vi "GeoData.vi"() -> ()   [LabVIEW 2017] (continued)
AL\tMontgomery County\tH1\n36131\t1101\tMontgomery\tAL\tMontgomery County\tH1\n36054\t1101\tMillbrook\tAL\tMontgomery County\tH1\n36109\t1101\tMontgomery\tAL\tMontgomery County\tH1\n36041\t1101\tHighland home\tAL\tMontgomery County\tH1\n36107\t1101\tMontgomery\tAL\tMontgomery County\tH1\n36121\t1101\tMontgomery\tAL\tMontgomery County\tH1\n36117\t1101\tMontgomery\tAL\tMontgomery County\tH1\n36120\t1101\tMontgomery\tAL\tMontgomery County\tH1\n36123\t1101\tMontgomery\tAL\tMontgomery County\tH1\n36064\t1101\tPike road\tAL\tMontgomery County\tH1\n36105\t1101\tMontgomery\tAL\tMontgomery County\tH1\n36106\t1101\tMontgomery\tAL\tMontgomery County\tH1\n36116\t1101\tMontgomery\tAL\tMontgomery County\tH1\n36119\t1101\tMontgomery\tAL\tMontgomery County\tH1\n36065\t1101\tPine level\tAL\tMontgomery County\tH1\n36036\t1101\tGrady\tAL\tMontgomery County\tH1\n36046\t1101\tLapine\tAL\tMontgomery County\tH1\n36057\t1101\tMount meigs\tAL\tMontgomery County\tH1\n35175\t1103\tUnion grove\tAL\tMorgan County\tH1\n35619\t1103\tDanville\tAL\tMorgan County\tH1\n35640\t1103\tHartselle\tAL\tMorgan County\tH1\n35602\t1103\tDecatur\tAL\tMorgan County\tH1\n35058\t1103\tCullman\tAL\tMorgan County\tH1\n35601\t1103\tDecatur\tAL\tMorgan County\tH1\n35087\t1103\tJoppa\tAL\tMorgan County\tH1\n35673\t1103\tTrinity\tAL\tMorgan County\tH1\n35775\t1103\tValhermoso springs\tAL\tMorgan County\tH1\n35603\t1103\tDecatur\tAL\tMorgan County\tH1\n35019\t1103\tBaileyton\tAL\tMorgan County\tH1\n35016\t1103\tArab\tAL\tMorgan County\tH1\n35754\t1103\tLaceys spring\tAL\tMorgan County\tH1\n35179\t1103\tVinemont\tAL\tMorgan County\tH1\n35621\t1103\tEva\tAL\tMorgan County\tH1\n35622\t1103\tFalkville\tAL\tMorgan County\tH1\n35670\t1103\tSomerville\tAL\tMorgan County\tH1\n36786\t1105\tUniontown\tAL\tPerry County\tH1\n36756\t1105\tMarion\tAL\tPerry County\tH1\n36773\t1105\tSafford\tAL\tPerry County\tH1\n36701\t1105\tSelma\tAL\tPerry County\tH1\n35042\t1105\tCentreville\tAL\tPerry County\tH1\n36765\t1105\tNewbern\tAL\tPerry County\tH1\n36728\t1105\tCatherine\tAL\tPerry County\tH1\n35034\t1105\tBrent\tAL\tPerry County\tH1\n36759\t1105\tMarion junction\tAL\tPerry County\tH1\n36793\t1105\tLawley\tAL\tPerry County\tH1\n35576\t1107\tMillport\tAL\tPickens County\tH1\n35466\t1107\tGordo\tAL\tPickens County\tH1\n35447\t1107\tCarrollton\tAL\tPickens County\tH1\n35471\t1107\tMc shan\tAL\tPickens County\tH1\n35481\t1107\tReform\tAL\tPickens County\tH1\n35442\t1107\tAliceville\tAL\tPickens County\tH1\n35461\t1107\tEthelsville\tAL\tPickens County\tH1\n35574\t1107\tKennedy\tAL\tPickens County\tH1\n35555\t1107\tFayette\tAL\tPickens County\tH1\n36082\t1109\tTroy\tAL\tPike County\tH1\n36079\t1109\tTroy\tAL\tPike County\tH1\n36081\t1109\tTroy\tAL\tPike County\tH1\n36049\t1109\tLuverne\tAL\tPike County\tH1\n36010\t1109\tBrundidge\tAL\tPike County\tH1\n36034\t1109\tGlenwood\tAL\tPike County\tH1\n36035\t1109\tGoshen\tAL\tPike County\tH1\n36005\t1109\tBanks\tAL\tPike County\tH1\n36264\t1111\tHeflin\tAL\tRandolph County\tH1\n36266\t1111\tLineville\tAL\tRandolph County\tH1\n36258\t1111\tDelta\tAL\tRandolph County\tH1\n36278\t1111\tWedowee\tAL\tRandolph County\tH1\n36263\t1111\tGraham\tAL\tRandolph County\tH1\n36276\t1111\tWadley\tAL\tRandolph County\tH1\n36280\t1111\tWoodland\tAL\tRandolph County\tH1\n36274\t1111\tRoanoke\tAL\tRandolph County\tH1\n36874\t1113\tSalem\tAL\tRussell County\tH1\n36871\t1113\tPittsview\tAL\tRussell County\tH1\n36877\t1113\tSmiths station\tAL\tRussell County\tH1\n36804\t1113\tOpelika\tAL\tRussell County\tH1\n36869\t1113\tPhenix city\tAL\tRussell County\tH1\n36860\t1113\tHurtsboro\tAL\tRussell County\tH1\n36875\t1113\tSeale\tAL\tRussell County\tH1\n36856\t1113\tFort mitchell\tAL\tRussell County\tH1\n36053\t1113\tMidway\tAL\tRussell County\tH1\n36858\t1113\tHatchechubbee\tAL\tRussell County\tH1\n36868\t1113\tPhenix city\tAL\tRussell County\tH1\n36851\t1113\tCottonton\tAL\tRussell County\tH1\n36027\t1113\tEufaula\tAL\tRussell County\tH1\n36867\t1113\tPhenix city\tAL\tRussell County\tH1\n36870\t1113\tPhenix city\tAL\tRussell County\tH1\n35135\t1115\tRiverside\tAL\tSt. Clair County\tH1\n35094\t1115\tLeeds\tAL\tSt. Clair County\tH1\n35146\t1115\tSpringville\tAL\tSt. Clair County\tH1\n35178\t1115\tVincent\tAL\tSt. Clair County\tH1\n35953\t1115\tAshville\tAL\tSt. Clair County\tH1\n35052\t1115\tCook springs\tAL\tSt. Clair County\tH1\n35112\t1115\tMargaret\tAL\tSt. Clair County\tH1\n35004\t1115\tMoody\tAL\tSt. Clair County\tH1\n35903\t1115\tGadsden\tAL\tSt. Clair County\tH1\n35173\t1115\tTrussville\tAL\tSt. Clair County\tH1\n35131\t1115\tRagland\tAL\tSt. Clair County\tH1\n35182\t1115\tWattsville\tAL\tSt. Clair County\tH1\n35133\t1115\tRemlap\tAL\tSt. Clair County\tH1\n35972\t1115\tGallant\tAL\tSt. Clair County\tH1\n35987\t1115\tSteele\tAL\tSt. Clair County\tH1\n35120\t1115\tOdenville\tAL\tSt. Clair County\tH1\n35125\t1115\tPell city\tAL\tSt. Clair County\tH1\n35128\t1115\tPell city\tAL\tSt. Clair County\tH1\n35121\t1115\tOneonta\tAL\tSt. Clair County\tH1\n35054\t1115\tCropwell\tAL\tSt. Clair County\tH1\n35906\t1115\tRainbow city\tAL\tSt. Clair County\tH1\n35022\t1117\tBessemer\tAL\tShelby County\tH1\n35115\t1117\tMontevallo\tAL\tShelby County\tH1\n35176\t1117\tVandiver\tAL\tShelby County\tH1\n35242\t1117\tBirmingham\tAL\tShelby County\tH1\n35244\t1117\tBirmingham\tAL\tShelby County\tH1\n35243\t1117\tBirmingham\tAL\tShelby County\tH1\n35051\t1117\tColumbiana\tAL\tShelby County\tH1\n35078\t1117\tHarpersville\tAL\tShelby County\tH1\n35094\t1117\tLeeds\tAL\tShelby County\tH1\n35114\t1117\tAlabaster\tAL\tShelby County\tH1\n35178\t1117\tVincent\tAL\tShelby County\tH1\n35216\t1117\tBirmingham\tAL\tShelby County\tH1\n35187\t1117\tWilton\tAL\tShelby County\tH1\n35238\t1117\tBirmingham\tAL\tShelby County\tH1\n35040\t1117\tCalera\tAL\tShelby County\tH1\n35137\t1117\tSaginaw\tAL\tShelby County\tH1\n35043\t1117\tChelsea\tAL\tShelby County\tH1\n35185\t1117\tWestover\tAL\tShelby County\tH1\n35007\t1117\tAlabaster\tAL\tShelby County\tH1\n35080\t1117\tHelena\tAL\tShelby County\tH1\n35147\t1117\tSterrett\tAL\tShelby County\tH1\n35124\t1117\tPelham\tAL\tShelby County\tH1\n35128\t1117\tPell city\tAL\tShelby County\tH1\n35035\t1117\tBrierfield\tAL\tShelby County\tH1\n35186\t1117\tWilsonville\tAL\tShelby County\tH1\n35143\t1117\tShelby\tAL\tShelby County\tH1\n36925\t1119\tYork\tAL\tSumter County\tH1\n36901\t1119\tBellamy\tAL\tSumter County\tH1\n36907\t1119\tCuba\tAL\tSumter County\tH1\n35464\t1119\tGainesville\tAL\tSumter County\tH1\n35442\t1119\tAliceville\tAL\tSumter County\tH1\n35470\t1119\tLivingston\tAL\tSumter County\tH1\n35459\t1119\tEmelle\tAL\tSumter County\tH1\n36912\t1119\tLisman\tAL\tSumter County\tH1\n35477\t1119\tPanola\tAL\tSumter County\tH1\n35460\t1119\tEpes\tAL\tSumter County\tH1\n36922\t1119\tWard\tAL\tSumter County\tH1\n35014\t1121\tAlpine\tAL\tTalladega County\tH1\n35151\t1121\tSylacauga\tAL\tTalladega County\tH1\n35032\t1121\tBon air\tAL\tTalladega County\tH1\n35096\t1121\tLincoln\tAL\tTalladega County\tH1\n35149\t1121\tSycamore\tAL\tTalladega County\tH1\n35150\t1121\tSylacauga\tAL\tTalladega County\tH1\n36260\t1121\tEastaboga\tAL\tTalladega County\tH1\n35072\t1121\tGoodwater\tAL\tTalladega County\tH1\n35160\t1121\tTalladega\tAL\tTalladega County\tH1\n36203\t1121\tOxford\tAL\tTalladega County\tH1\n35044\t1121\tChildersburg\tAL\tTalladega County\tH1\n36268\t1121\tMunford\tAL\tTalladega County\tH1\n35082\t1121\tHollins\tAL\tTalladega County\tH1\n36251\t1123\tAshland\tAL\tTallapoosa County\tH1\n36849\t1123\tAuburn university\tAL\tTallapoosa County\tH1\n35010\t1123\tAlexander city\tAL\tTallapoosa County\tH1\n36078\t1123\tTallassee\tAL\tTallapoosa County\tH1\n35089\t1123\tKellyton\tAL\tTallapoosa County\tH1\n36853\t1123\tDadeville\tAL\tTallapoosa County\tH1\n36256\t1123\tDaviston\tAL\tTallapoosa County\tH1\n36850\t1123\tCamp hill\tAL\tTallapoosa County\tH1\n36879\t1123\tWaverly\tAL\tTallapoosa County\tH1\n36255\t1123\tCragford\tAL\tTallapoosa County\tH1\n35072\t1123\tGoodwater\tAL\tTallapoosa County\tH1\n36866\t1123\tNotasulga\tAL\tTallapoosa County\tH1\n36276\t1123\tWadley\tAL\tTallapoosa County\tH1\n36861\t1123\tJacksons gap\tAL\tTallapoosa County\tH1\n35184\t1125\tWest blocton\tAL\tTuscaloosa County\tH1\n35490\t1125\tVance\tAL\tTuscaloosa County\tH1\n35546\t1125\tBerry\tAL\tTuscaloosa County\tH1\n35453\t1125\tCottondale\tAL\tTuscaloosa County\tH1\n35458\t1125\tElrod\tAL\tTuscaloosa County\tH1\n35466\t1125\tGordo\tAL\tTuscaloosa County\tH1\n35475\t1125\tNorthport\tAL\tTuscaloosa County\tH1\n35480\t1125\tRalph\tAL\tTuscaloosa County\tH1\n35440\t1125\tAbernant\tAL\tTuscaloosa County\tH1\n35579\t1125\tOakman\tAL\tTuscaloosa County\tH1\n35486\t1125\tTuscaloosa\tAL\tTuscaloosa County\tH1\n35444\t1125\tBrookwood\tAL\tTuscaloosa County\tH1\n35111\t1125\tMc calla\tAL\tTuscaloosa County\tH1\n35473\t1125\tNorthport\tAL\tTuscaloosa County\tH1\n35476\t1125\tNorthport\tAL\tTuscaloosa County\tH1\n35452\t1125\tCoker\tAL\tTuscaloosa County\tH1\n35456\t1125\tDuncanville\tAL\tTuscaloosa County\tH1\n35403\t1125\tTuscaloosa\tAL\tTuscaloosa County\tH1\n35402\t1125\tTuscaloosa\tAL\tTuscaloosa County\tH1\n35006\t1125\tAdger\tAL\tTuscaloosa County\tH1\n35457\t1125\tEchola\tAL\tTuscaloosa County\tH1\n35449\t1125\tCoaling\tAL\tTuscaloosa County\tH1\n35468\t1125\tKellerman\tAL\tTuscaloosa County\tH1\n35406\t1125\tTuscaloosa\tAL\tTuscaloosa County\tH1\n35474\t1125\tMoundville\tAL\tTuscaloosa County\tH1\n35407\t1125\tTuscaloosa\tAL\tTuscaloosa County\tH1\n35463\t1125\tFosters\tAL\tTuscaloosa County\tH1\n35574\t1125\tKennedy\tAL\tTuscaloosa County\tH1\n35469\t1125\tKnoxville\tAL\tTuscaloosa County\tH1\n35188\t1125\tWoodstock\tAL\tTuscaloosa County\tH1\n35555\t1125\tFayette\tAL\tTuscaloosa County\tH1\n35401\t1125\tTuscaloosa\tAL\tTuscaloosa County\tH1\n35404\t1125\tTuscaloosa\tAL\tTuscaloosa County\tH1\n35405\t1125\tTuscaloosa\tAL\tTuscaloosa County\tH1\n35446\t1125\tBuhl\tAL\tTuscaloosa County\tH1\n35482\t1125\tSamantha\tAL\tTuscaloosa County\tH1\n35478\t1125\tPeterson\tAL\tTuscaloosa County\tH1\n35130\t1127\tQuinton\tAL\tWalker County\tH1\n35554\t1127\tEldridge\tAL\tWalker County\tH1\n35546\t1127\tBerry\tAL\tWalker County\tH1\n35549\t1127\tCarbon hill\tAL\tWalker County\tH1\n35063\t1127\tEmpire\tAL\tWalker County\tH1\n35033\t1127\tBremen\tAL\tWalker County\tH1\n35579\t1127\tOakman\tAL\tWalker County\tH1\n35573\t1127\tKansas\tAL\tWalker County\tH1\n35006\t1127\tAdger\tAL\tWalker County\tH1\n35580\t1127\tParrish\tAL\tWalker County\tH1\n35578\t1127\tNauvoo\tAL\tWalker County\tH1\n35148\t1127\tSumiton\tAL\tWalker County\tH1\n35502\t1127\tJasper\tAL\tWalker County\tH1\n35587\t1127\tTownley\tAL\tWalker County\tH1\n35560\t1127\tGoodsprings\tAL\tWalker County\tH1\n35062\t1127\tDora\tAL\tWalker County\tH1\n35503\t1127\tJasper\tAL\tWalker County\tH1\n35504\t1127\tJasper\tAL\tWalker County\tH1\n35501\t1127\tJasper\tAL\tWalker County\tH1\n35550\t1127\tCordova\tAL\tWalker County\tH1\n35584\t1127\tSipsey\tAL\tWalker County\tH1\n35038\t1127\tBurnwell\tAL\tWalker County\tH1\n36529\t1129\tDeer park\tAL\tWashington County\tH1\n36581\t1129\tSunflower\tAL\tWashington County\tH1\n36569\t1129\tSaint stephens\tAL\tWashington County\tH1\n36583\t1129\tTibbie\tAL\tWashington County\tH1\n36538\t1129\tFrankville\tAL\tWashington County\tH1\n36518\t1129\tChatom\tAL\tWashington County\tH1\n36539\t1129\tFruitdale\tAL\tWashington County\tH1\n36513\t1129\tCalvert\tAL\tWashington County\tH1\n36556\t1129\tMalcolm\tAL\tWashington County\tH1\n36584\t1129\tVinegar bend\tAL\tWashington County\tH1\n36553\t1129\tMc intosh\tAL\tWashington County\tH1\n36548\t1129\tLeroy\tAL\tWashington County\tH1\n36522\t1129\tCitronelle\tAL\tWashington County\tH1\n36585\t1129\tWagarville\tAL\tWashington County\tH1\n36558\t1129\tMillry\tAL\tWashington County\tH1\n36722\t1131\tArlington\tAL\tWilcox County\tH1\n36751\t1131\tLower peach tree\tAL\tWilcox County\tH1\n36741\t1131\tFurman\tAL\tWilcox County\tH1\n36783\t1131\tThomaston\tAL\tWilcox County\tH1\n36720\t1131\tAlberta\tAL\tWilcox County\tH1\n36726\t1131\tCamden\tAL\tWilcox County\tH1\n36728\t1131\tCatherine\tAL\tWilcox County\tH1\n36766\t1131\tOak hill\tAL\tWilcox County\tH1\n36435\t1131\tCoy\tAL\tWilcox County\tH1\n36769\t1131\tPine hill\tAL\tWilcox County\tH1\n36784\t1131\tThomasville\tAL\tWilcox County\tH1\n36030\t1131\tForest home\tAL\tWilcox County\tH1\n36761\t1131\tMinter\tAL\tWilcox County\tH1\n36753\t1131\tMc williams\tAL\tWilcox County\tH1\n36768\t1131\tPine apple\tAL\tWilcox County\tH1\n36723\t1131\tBoykin\tAL\tWilcox County\tH1\n35541\t1133\tArley\tAL\tWinston County\tH1\n35572\t1133\tHouston\tAL\tWinston County\tH1\n35057\t1133\tCullman\tAL\tWinston County\tH1\n35553\t1133\tDouble springs\tAL\tWinston County\tH1\n35565\t1133\tHaleyville\tAL\tWinston County\tH1\n35578\t1133\tNauvoo\tAL\tWinston County\tH1\n35551\t1133\tDelmar\tAL\tWinston County\tH1\n35098\t1133\tLogan\tAL\tWinston County\tH1\n35575\t1133\tLynn\tAL\tWinston County\tH1\n35053\t1133\tCrane hill\tAL\tWinston County\tH1\n35577\t1133\tNatural bridge\tAL\tWinston County\tH1\n35179\t1133\tVinemont\tAL\tWinston County\tH1\n35503\t1133\tJasper\tAL\tWinston County\tH1\n35540\t1133\tAddison\tAL\tWinston County\tH1\n99661\t2013\tSand point\tAK\tAleutians East Borough\tH1\n99612\t2013\tKing cove\tAK\tAleutians East Borough\tH1\n99553\t2013\tAkutan\tAK\tAleutians East Borough\tH1\n99571\t2013\tCold bay\tAK\tAleutians East Borough\tH1\n99583\t2013\tFalse pass\tAK\tAleutians East Borough\tH1\n99692\t2016\tDutch harbor\tAK\tAleutians West Census Area\tH5\n99638\t2016\tNikolski\tAK\tAleutians West Census Area\tH5\n99660\t2016\tSaint paul island\tAK\tAleutians West Census Area\tH5\n99685\t2016\tUnalaska\tAK\tAleutians West Census Area\tH5\n99547\t2016\tAtka\tAK\tAleutians West Census Area\tH5\n99591\t2016\tSaint george island\tAK\tAleutians West Census Area\tH5\n99546\t2016\tAdak\tAK\tAleutians West Census Area\tH5\n99523\t2020\tAnchorage\tAK\tAnchorage Municipality\tH6\n99587\t2020\tGirdwood\tAK\tAnchorage Municipality\tH6\n99567\t2020\tChugiak\tAK\tAnchorage Municipality\tH6\n99505\t2020\tJber\tAK\tAnchorage Municipality\tH6\n99521\t2020\tAnchorage\tAK\tAnchorage Municipality\tH6\n99529\t2020\tAnchorage\tAK\tAnchorage Municipality\tH6\n99520\t2020\tAnchorage\tAK\tAnchorage Municipality\tH6\n99506\t2020\tJber\tAK\tAnchorage Municipality\tH6\n99511\t2020\tAnchorage\tAK\tAnchorage Municipality\tH6\n99540\t2020\tIndian\tAK\tAnchorage Municipality\tH6\n99515\t2020\tAnchorage\tAK\tAnchorage Municipality\tH6\n99522\t2020\tAnchorage\tAK\tAnchorage Municipality\tH6\n99577\t2020\tEagle river\tAK\tAnchorage Municipality\tH6\n99510\t2020\tAnchorage\tAK\tAnchorage Municipality\tH6\n99524\t2020\tAnchorage\tAK\tAnchorage Municipality\tH6\n99518\t2020\tAnchorage\tAK\tAnchorage Municipality\tH6\n99502\t2020\tAnchorage\tAK\tAnchorage Municipality\tH6\n99519\t2020\tAnchorage\tAK\tAnchorage Municipality\tH6\n99501\t2020\tAnchorage\tAK\tAnchorage Municipality\tH6\n99503\t2020\tAnchorage\tAK\tAnchorage Municipality\tH6\n99507\t2020\tAnchorage\tAK\tAnchorage Municipality\tH6\n99509\t2020\tAnchorage\tAK\tAnchorage Municipality\tH6\n99516\t2020\tAnchorage\tAK\tAnchorage Municipality\tH6\n99514\t2020\tAnchorage\tAK\tAnchorage Municipality\tH6\n99599\t2020\tAnchorage\tAK\tAnchorage Municipality\tH6\n99508\t2020\tAnchorage\tAK\tAnchorage Municipality\tH6\n99517\t2020\tAnchorage\tAK\tAnchorage Municipality\tH6\n99504\t2020\tAnchorage\tAK\tAnchorage Municipality\tH6\n99513\t2020\tAnchorage\tAK\tAnchorage Municipality\tH6\n99530\t2020\tAnchorage\tAK\tAnchorage Municipality\tH6\n99614\t2050\tKipnuk\tAK\tBethel Census Area\tH5\n99668\t2050\tSleetmute\tAK\tBethel Census Area\tH5\n99679\t2050\tTuluksak\tAK\tBethel Census Area\tH5\n99545\t2050\tKongiganak\tAK\tBethel Census Area\tH5\n99655\t2050\tQuinhagak\tAK\tBethel Census Area\tH5\n99589\t2050\tGoodnews bay\tAK\tBethel Census Area\tH5\n99634\t2050\tNapakiak\tAK\tBethel Census Area\tH5\n99656\t2050\tRed devil\tAK\tBethel Census Area\tH5\n99626\t2050\tLower kalskag\tAK\tBethel Census Area\tH5\n99681\t2050\tTununak\tAK\tBethel Census Area\tH5\n99651\t2050\tPlatinum\tAK\tBethel Census Area\tH5\n99637\t2050\tToksook bay\tAK\tBethel Census Area\tH5\n99622\t2050\tKwigillingok\tAK\tBethel Census Area\tH5\n99559\t2050\tBethel\tAK\tBethel Census Area\tH5\n99607\t2050\tKalskag\tAK\tBethel Census Area\tH5\n99557\t2050\tAniak\tAK\tBethel Census Area\tH5\n99630\t2050\tMekoryuk\tAK\tBethel Census Area\tH5\n99561\t2050\tChefornak\tAK\tBethel Census Area\tH5\n99690\t2050\tNightmute\tAK\tBethel Census Area\tH5\n99551\t2050\tAkiachak\tAK\tBethel Census Area\tH5\n99575\t2050\tCrooked creek\tAK\tBethel Census Area\tH5\n99578\t2050\tEek\tAK\tBethel Census Area\tH5\n99609\t2050\tKasigluk\tAK\tBethel Census Area\tH5\n99552\t2050\tAkiak\tAK\tBethel Census Area\tH5\n99621\t2050\tKwethluk\tAK\tBethel Census Area\tH5\n99680\t2050\tTuntutuliak\tAK\tBethel Census Area\tH5\n99641\t2050\tNunapitchuk\tAK\tBethel Census Area\tH5\n99670\t2060\tSouth naknek\tAK\tBristol Bay Borough\tH1\n99633\t2060\tNaknek\tAK\tBristol Bay Borough\tH1\n99613\t2060\tKing salmon\tAK\tBristol Bay Borough\tH1\n99744\t2068\tAnderson\tAK\tDenali Borough\tH1\n99755\t2068\tDenali national park\tAK\tDenali Borough\tH1\n99729\t2068\tCantwell\tAK\tDenali Borough\tH1\n99743\t2068\tHealy\tAK\tDenali Borough\tH1\n99628\t2070\tManokotak\tAK\tDillingham Census Area\tH5\n99555\t2070\tAleknagik\tAK\tDillingham Census Area\tH5\n99678\t2070\tTogiak\tAK\tDillingham Census Area\tH5\n99576\t2070\tDillingham\tAK\tDillingham Census Area\tH5\n99636\t2070\tNew stuyahok\tAK\tDillingham Census Area\tH5\n99580\t2070\tEkwok\tAK\tDillingham Census Area\tH5\n99569\t2070\tClarks point\tAK\tDillingham Census Area\tH5\n99712\t2090\tFairbanks\tAK\tFairbanks North Star Borough\tH1\n99709\t2090\tFairbanks\tAK\tFairbanks North Star Borough\tH1\n99707\t2090\tFairbanks\tAK\tFairbanks North Star Borough\tH1\n99702\t2090\tEielson afb\tAK\tFairbanks North Star Borough\tH1\n99775\t2090\tFairbanks\tAK\tFairbanks North Star Borough\tH1\n99706\t2090\tFairbanks\tAK\tFairbanks North Star Borough\tH1\n99790\t2090\tFairbanks\tAK\tFairbanks North Star Borough\tH1\n99714\t2090\tSalcha\tAK\tFairbanks North Star Borough\tH1\n99708\t2090\tFairbanks\tAK\tFairbanks North Star Borough\tH1\n99725\t2090\tEster\tAK\tFairbanks North Star Borough\tH1\n99701\t2090\tFairbanks\tAK\tFairbanks North Star Borough\tH1\n99703\t2090\tFort wainwright\tAK\tFairbanks North Star Borough\tH1\n99705\t2090\tNorth pole\tAK\tFairbanks North Star Borough\tH1\n99827\t2100\tHaines\tAK\tHaines Borough\tH1\n99825\t2105\tElfin cove\tAK\tHoonah-Angoon Census Area\tH5\n99832\t2105\tPelican\tAK\tHoonah-Angoon Census Area\tH5\n99829\t2105\tHoonah\tAK\tHoonah-Angoon Census Area\tH5\n99841\t2105\tTenakee springs\tAK\tHoonah-Angoon Census Area\tH5\n99826\t2105\tGustavus\tAK\tHoonah-Angoon Census Area\tH5\n99820\t2105\tAngoon\tAK\tHoonah-Angoon Census Area\tH5\n99801\t2110\tJuneau\tAK\tJuneau City and Borough\tH6\n99824\t2110\tDouglas\tAK\tJuneau City and Borough\tH6\n99811\t2110\tJuneau\tAK\tJuneau City and Borough\tH6\n99672\t2122\tSterling\tAK\tKenai Peninsula Borough\tH1\n99682\t2122\tTyonek\tAK\tKenai Peninsula Borough\tH1\n99639\t2122\tNinilchik\tAK\tKenai Peninsula Borough\tH1\n99605\t2122\tHope\tAK\tKenai Peninsula Borough\tH1\n99669\t2122\tSoldotna\tAK\tKenai Peninsula Borough\tH1\n99664\t2122\tSeward\tAK\tKenai Peninsula Borough\tH1\n99568\t2122\tClam gulch\tAK\tKenai Peninsula Borough\tH1\n99635\t2122\tNikiski\tAK\tKenai Peninsula Borough\tH1\n99603\t2122\tHomer\tAK\tKenai Peninsula Borough\tH1\n99556\t2122\tAnchor point\tAK\tKenai Peninsula Borough\tH1\n99611\t2122\tKenai\tAK\tKenai Peninsula Borough\tH1\n99572\t2122\tCooper landing\tAK\tKenai Peninsula Borough\tH1\n99631\t2122\tMoose pass\tAK\tKenai Peninsula Borough\tH1\n99610\t2122\tKasilof\tAK\tKenai Peninsula Borough\tH1\n99663\t2122\tSeldovia\tAK\tKenai Peninsula Borough\tH1\n99901\t2130\tKetchikan\tAK\tKetchikan Gateway Borough\tH1\n99928\t2130\tWard cove\tAK\tKetchikan Gateway Borough\tH1\n99643\t2150\tOld harbor\tAK\tKodiak Island Borough\tH1\n99550\t2150\tPort lions\tAK\tKodiak Island Borough\tH1\n99615\t2150\tKodiak\tAK\tKodiak Island Borough\tH1\n99624\t2150\tLarsen bay\tAK\tKodiak Island Borough\tH1\n99608\t2150\tKarluk\tAK\tKodiak Island Borough\tH1\n99644\t2150\tOuzinkie\tAK\tKodiak Island Borough\tH1\n99625\t2164\tLevelock\tAK\tLake and Peninsula Borough\tH1\n99548\t2164\tChignik lake\tAK\tLake and Peninsula Borough\tH1\n99649\t2164\tPilot point\tAK\tLake and Peninsula Borough\tH1\n99640\t2164\tNondalton\tAK\tLake and Peninsula Borough\tH1\n99653\t2164\tPort alsworth\tAK\tLake and Peninsula Borough\tH1\n99549\t2164\tPort heiden\tAK\tLake and Peninsula Borough\tH1\n99565\t2164\tChignik lagoon\tAK\tLake and Peninsula Borough\tH1\n99579\t2164\tEgegik\tAK\tLake and Peninsula Borough\tH1\n99648\t2164\tPerryville\tAK\tLake and Peninsula Borough\tH1\n99564\t2164\tChignik\tAK\tLake and Peninsula Borough\tH1\n99606\t2164\tIliamna\tAK\tLake and Peninsula Borough\tH1\n99647\t2164\tPedro bay\tAK\tLake and Peninsula Borough\tH1\n99654\t2170\tWasilla\tAK\tMatanuska-Susitna Borough\tH1\n99623\t2170\tWasilla\tAK\tMatanuska-Susitna Borough\tH1\n99645\t2170\tPalmer\tAK\tMatanuska-Susitna Borough\tH1\n99683\t2170\tTrapper creek\tAK\tMatanuska-Susitna Borough\tH1\n99674\t2170\tSutton\tAK\tMatanuska-Susitna Borough\tH1\n99676\t2170\tTalkeetna\tAK\tMatanuska-Susitna Borough\tH1\n99667\t2170\tSkwentna\tAK\tMatanuska-Susitna Borough\tH1\n99687\t2170\tWasilla\tAK\tMatanuska-Susitna Borough\tH1\n99652\t2170\tBig lake\tAK\tMatanuska-Susitna Borough\tH1\n99688\t2170\tWillow\tAK\tMatanuska-Susitna Borough\tH1\n99694\t2170\tHouston\tAK\tMatanuska-Susitna Borough\tH1\n99769\t2180\tSavoonga\tAK\tNome Census Area\tH5\n99684\t2180\tUnalakleet\tAK\tNome Census Area\tH5\n99784\t2180\tWhite mountain\tAK\tNome Census Area\tH5\n99671\t2180\tStebbins\tAK\tNome Census Area\tH5\n99739\t2180\tElim\tAK\tNome Census Area\tH5\n99778\t2180\tTeller\tAK\tNome Census Area\tH5\n99742\t2180\tGambell\tAK\tNome Census Area\tH5\n99753\t2180\tKoyuk\tAK\tNome Census Area\tH5\n99772\t2180\tShishmaref\tAK\tNome Census Area\tH5\n99783\t2180\tWales\tAK\tNome Census Area\tH5\n99762\t2180\tNome\tAK\tNome Census Area\tH5\n99771\t2180\tShaktoolik\tAK\tNome Census Area\tH5\n99785\t2180\tBrevig mission\tAK\tNome Census Area\tH5\n99659\t2180\tSaint michael\tAK\tNome Census Area\tH5\n99747\t2185\tKaktovik\tAK\tNorth Slope Borough\tH1\n99782\t2185\tWainwright\tAK\tNorth Slope Borough\tH1\n99734\t2185\tPrudhoe bay\tAK\tNorth Slope Borough\tH1\n99789\t2185\tNuiqsut\tAK\tNorth Slope Borough\tH1\n99759\t2185\tPoint lay\tAK\tNorth Slope Borough\tH1\n99723\t2185\tBarrow\tAK\tNorth Slope Borough\tH1\n99766\t2185\tPoint hope\tAK\tNorth Slope Borough\tH1\n99721\t2185\tAnaktuvuk pass\tAK\tNorth Slope Borough\tH1\n99791\t2185\tAtqasuk\tAK\tNorth Slope Borough\tH1\n99749\t2188\tKiana\tAK\tNorthwest Arctic Borough\tH1\n99727\t2188\tBuckland\tAK\tNorthwest Arctic Borough\tH1\n99750\t2188\tKivalina\tAK\tNorthwest Arctic Borough\tH1\n99770\t2188\tSelawik\tAK\tNorthwest Arctic Borough\tH1\n99773\t2188\tShungnak\tAK\tNorthwest Arctic Borough\tH1\n99763\t2188\tNoorvik\tAK\tNorthwest Arctic Borough\tH1\n99761\t2188\tNoatak\tAK\tNorthwest Arctic Borough\tH1\n99786\t2188\tAmbler\tAK\tNorthwest Arctic Borough\tH1\n99752\t2188\tKotzebue\tAK\tNorthwest Arctic Borough\tH1\n99736\t2188\tDeering\tAK\tNorthwest Arctic Borough\tH1\n99751\t2188\tKobuk\tAK\tNorthwest Arctic Borough\tH1\n99836\t2195\tPort alexander\tAK\tPetersburg Census Area\tH5\n99830\t2195\tKake\tAK\tPetersburg Census Area\tH5\n99833\t2195\tPetersburg\tAK\tPetersburg Census Area\tH5\n99923\t2198\tHyder\tAK\tPrince of Wales-Hyder Census Area\tH5\n99918\t2198\tCoffman cove\tAK\tPrince of Wales-Hyder Census Area\tH5\n99922\t2198\tHydaburg\tAK\tPrince of Wales-Hyder Census Area\tH5\n99921\t2198\tCraig\tAK\tPrince of Wales-Hyder Census Area\tH5\n99927\t2198\tPoint baker\tAK\tPrince of Wales-Hyder Census Area\tH5\n99919\t2198\tThorne bay\tAK\tPrince of Wales-Hyder Census Area\tH5\n99925\t2198\tKlawock\tAK\tPrince of Wales-Hyder Census Area\tH5\n99926\t2198\tMetlakatla\tAK\tPrince of Wales-Hyder Census Area\tH5\n99835\t2220\tSitka\tAK\tSitka City and Borough\tH6\n99840\t2230\tSkagway\tAK\tSkagway Municipality\tH1\n99738\t2240\tEagle\tAK\tSoutheast Fairbanks Census Area\tH5\n99737\t2240\tDelta junction\tAK\tSoutheast Fairbanks Census Area\tH5\n99780\t2240\tTok\tAK\tSoutheast Fairbanks Census Area\tH5\n99732\t2240\tChicken\tAK\tSoutheast Fairbanks Census Area\tH5\n99764\t2240\tNorthway\tAK\tSoutheast Fairbanks Census Area\tH5\n99776\t2240\tTanacross\tAK\tSoutheast Fairbanks Census Area\tH5\n99731\t2240\tFort greely\tAK\tSoutheast Fairbanks Census Area\tH5\n99588\t2261\tGlennallen\tAK\tValdez-Cordova Census Area\tH5\n99693\t2261\tWhittier\tAK\tValdez-Cordova Census Area\tH5\n99566\t2261\tChitina\tAK\tValdez-Cordova Census Area\tH5\n99586\t2261\tGakona\tAK\tValdez-Cordova Census Area\tH5\n99677\t2261\tTatitlek\tAK\tValdez-Cordova Census Area\tH5\n99686\t2261\tValdez\tAK\tValdez-Cordova Census Area\tH5\n99573\t2261\tCopper center\tAK\tValdez-Cordova Census Area\tH5\n99574\t2261\tCordova\tAK\tValdez-Cordova Census Area\tH5\n99903\t2275\tMeyers chuck\tAK\tWrangell City and Borough\tH1\n99929\t2275\tWrangell\tAK\tWrangell City and Borough\tH1\n99689\t2282\tYakutat\tAK\tYakutat City and Borough\tH1\n99627\t2290\tMc grath\tAK\tYukon-Koyukuk Census Area\tH5\n99760\t2290\tNenana\tAK\tYukon-Koyukuk Census Area\tH5\n99754\t2290\tKoyukuk\tAK\tYukon-Koyukuk Census Area\tH5\n99675\t2290\tTakotna\tAK\tYukon-Koyukuk Census Area\tH5\n99558\t2290\tAnvik\tAK\tYukon-Koyukuk Census Area\tH5\n99665\t2290\tShageluk\tAK\tYukon-Koyukuk Census Area\tH5\n99765\t2290\tNulato\tAK\tYukon-Koyukuk Census Area\tH5\n99768\t2290\tRuby\tAK\tYukon-Koyukuk Census Area\tH5\n99757\t2290\tLake minchumina\tAK\tYukon-Koyukuk Census Area\tH5\n99745\t2290\tHughes\tAK\tYukon-Koyukuk Census Area\tH5\n99704\t2290\tClear\tAK\tYukon-Koyukuk Census Area\tH5\n99720\t2290\tAllakaket\tAK\tYukon-Koyukuk Census Area\tH5\n99741\t2290\tGalena\tAK\tYukon-Koyukuk Census Area\tH5\n99746\t2290\tHuslia\tAK\tYukon-Koyukuk Census Area\tH5\n99733\t2290\tCircle\tAK\tYukon-Koyukuk Census Area\tH5\n99777\t2290\tTanana\tAK\tYukon-Koyukuk Census Area\tH5\n99722\t2290\tArctic village\tAK\tYukon-Koyukuk Census Area\tH5\n99730\t2290\tCentral\tAK\tYukon-Koyukuk Census Area\tH5\n99788\t2290\tChalkyitsik\tAK\tYukon-Koyukuk Census Area\tH5\n99590\t2290\tGrayling\tAK\tYukon-Koyukuk Census Area\tH5\n99740\t2290\tFort yukon\tAK\tYukon-Koyukuk Census Area\tH5\n99756\t2290\tManley hot springs\tAK\tYukon-Koyukuk Census Area\tH5\n99691\t2290\tNikolai\tAK\tYukon-Koyukuk Census Area\tH5\n99758\t2290\tMinto\tAK\tYukon-Koyukuk Census Area\tH5\n99774\t2290\tStevens village\tAK\tYukon-Koyukuk Census Area\tH5\n99748\t2290\tKaltag\tAK\tYukon-Koyukuk Census Area\tH5\n99602\t2290\tHoly cross\tAK\tYukon-Koyukuk Census Area\tH5\n99726\t2290\tBettles field\tAK\tYukon-Koyukuk Census Area\tH5\n99781\t2290\tVenetie\tAK\tYukon-Koyukuk Census Area\tH5\n99767\t2290\tRampart\tAK\tYukon-Koyukuk Census Area\tH5\n99724\t2290\tBeaver\tAK\tYukon-Koyukuk Census Area\tH5\n86556\t4001\tTsaile\tAZ\tApache County\tH1\n85901\t4001\tShow low\tAZ\tApache County\tH1\n86504\t4001\tFort defiance\tAZ\tApache County\tH1\n85920\t4001\tAlpine\tAZ\tApache County\tH1\n86506\t4001\tHouck\tAZ\tApache County\tH1\n85932\t4001\tNutrioso\tAZ\tApache County\tH1\n86502\t4001\tChambers\tAZ\tApache County\tH1\n86545\t4001\tRock point\tAZ\tApache County\tH1\n85924\t4001\tConcho\tAZ\tApache County\tH1\n85940\t4001\tVernon\tAZ\tApache County\tH1\n86503\t4001\tChinle\tAZ\tApache County\tH1\n85938\t4001\tSpringerville\tAZ\tApache County\tH1\n85927\t4001\tGreer\tAZ\tApache County\tH1\n85930\t4001\tMcnary\tAZ\tApache County\tH1\n86505\t4001\tGanado\tAZ\tApache County\tH1\n85937\t4001\tSnowflake\tAZ\tApache County\tH1\n86508\t4001\tLupton\tAZ\tApache County\tH1\n86535\t4001\tDennehotso\tAZ\tApache County\tH1\n86512\t4001\tSanders\tAZ\tApache County\tH1\n86514\t4001\tTeec nos pos\tAZ\tApache County\tH1\n86511\t4001\tSaint michaels\tAZ\tApache County\tH1\n86028\t4001\tPetrified forest natl pk\tAZ\tApache County\tH1\n86507\t4001\tLukachukai\tAZ\tApache County\tH1\n86544\t4001\tRed valley\tAZ\tApache County\tH1\n86540\t4001\tNazlini\tAZ\tApache County\tH1\n86538\t4001\tMany farms\tAZ\tApache County\tH1\n85925\t4001\tEagar\tAZ\tApache County\tH1\n86515\t4001\tWindow rock\tAZ\tApache County\tH1\n86547\t4001\tRound rock\tAZ\tApache County\tH1\n85936\t4001\tSaint johns\tAZ\tApache County\tH1\n85617\t4003\tMc neal\tAZ\tCochise County\tH1\n85636\t4003\tSierra vista\tAZ\tCochise County\tH1\n85616\t4003\tHuachuca city\tAZ\tCochise County\tH1\n85606\t4003\tCochise\tAZ\tCochise County\tH1\n85627\t4003\tPomerene\tAZ\tCochise County\tH1\n85615\t4003\tHereford\tAZ\tCochise County\tH1\n85625\t4003\tPearce\tAZ\tCochise County\tH1\n85605\t4003\tBowie\tAZ\tCochise County\tH1\n85635\t4003\tSierra vista\tAZ\tCochise County\tH1\n85650\t4003\tSierra vista\tAZ\tCochise County\tH1\n85608\t4003\tDouglas\tAZ\tCochise County\tH1\n85610\t4003\tElfrida\tAZ\tCochise County\tH1\n85602\t4003\tBenson\tAZ\tCochise County\tH1\n85643\t4003\tWillcox\tAZ\tCochise County\tH1\n85620\t4003\tNaco\tAZ\tCochise County\tH1\n85626\t4003\tPirtleville\tAZ\tCochise County\tH1\n85638\t4003\tTombstone\tAZ\tCochise County\tH1\n85603\t4003\tBisbee\tAZ\tCochise County\tH1\n85632\t4003\tSan simon\tAZ\tCochise County\tH1\n85624\t4003\tPatagonia\tAZ\tCochise County\tH1\n85630\t4003\tSaint david\tAZ\tCochise County\tH1\n85607\t4003\tDouglas\tAZ\tCochise County\tH1\n85613\t4003\tFort huachuca\tAZ\tCochise County\tH1\n85611\t4003\tElgin\tAZ\tCochise County\tH1\n85609\t4003\tDragoon\tAZ\tCochise County\tH1\n86002\t4005\tFlagstaff\tAZ\tCoconino County\tH1\n86003\t4005\tFlagstaff\tAZ\tCoconino County\tH1\n86024\t4005\tHappy jack\tAZ\tCoconino County\tH1\n86005\t4005\tFlagstaff\tAZ\tCoconino County\tH1\n86044\t4005\tTonalea\tAZ\tCoconino County\tH1\n86017\t4005\tMunds park\tAZ\tCoconino County\tH1\n86047\t4005\tWinslow\tAZ\tCoconino County\tH1\n86336\t4005\tSedona\tAZ\tCoconino County\tH1\n86022\t4005\tFredonia\tAZ\tCoconino County\tH1\n86020\t4005\tCameron\tAZ\tCoconino County\tH1\n86023\t4005\tGrand canyon\tAZ\tCoconino County\tH1\n85928\t4005\tHeber\tAZ\tCoconino County\tH1\n86038\t4005\tMormon lake\tAZ\tCoconino County\tH1\n86053\t4005\tKaibeto\tAZ\tCoconino County\tH1\n85931\t4005\tForest lakes\tAZ\tCoconino County\tH1\n86011\t4005\tFlagstaff\tAZ\tCoconino County\tH1\n86015\t4005\tBellemont\tAZ\tCoconino County\tH1\n86040\t4005\tPage\tAZ\tCoconino County\tH1\n86339\t4005\tSedona\tAZ\tCoconino County\tH1\n86046\t4005\tWilliams\tAZ\tCoconino County\tH1\n86036\t4005\tMarble canyon\tAZ\tCoconino County\tH1\n86045\t4005\tTuba city\tAZ\tCoconino County\tH1\n86018\t4005\tParks\tAZ\tCoconino County\tH1\n86052\t4005\tNorth rim\tAZ\tCoconino County\tH1\n86001\t4005\tFlagstaff\tAZ\tCoconino County\tH1\n86004\t4005\tFlagstaff\tAZ\tCoconino County\tH1\n86435\t4005\tSupai\tAZ\tCoconino County\tH1\n86016\t4005\tGray mountain\tAZ\tCoconino County\tH1\n85541\t4007\tPayson\tAZ\tGila County\tH1\n85192\t4007\tWinkelman\tAZ\tGila County\tH1\n85545\t4007\tRoosevelt\tAZ\tGila County\tH1\n85135\t4007\tHayden\tAZ\tGila County\tH1\n85554\t4007\tYoung\tAZ\tGila County\tH1\n85544\t4007\tPine\tAZ\tGila County\tH1\n85501\t4007\tGlobe\tAZ\tGila County\tH1\n85547\t4007\tPayson\tAZ\tGila County\tH1\n85532\t4007\tClaypool\tAZ\tGila County\tH1\n85539\t4007\tMiami\tAZ\tGila County\tH1\n85542\t4007\tPeridot\tAZ\tGila County\tH1\n85553\t4007\tTonto basin\tAZ\tGila County\tH1\n85543\t4009\tPima\tAZ\tGraham County\tH1\n85551\t4009\tSolomon\tAZ\tGraham County\tH1\n85535\t4009\tEden\tAZ\tGraham County\tH1\n85550\t4009\tSan carlos\tAZ\tGraham County\tH1\n85531\t4009\tCentral\tAZ\tGraham County\tH1\n85536\t4009\tFort thomas\tAZ\tGraham County\tH1\n85546\t4009\tSafford\tAZ\tGraham County\tH1\n85552\t4009\tThatcher\tAZ\tGraham County\tH1\n85643\t4009\tWillcox\tAZ\tGraham County\tH1\n85548\t4009\tSafford\tAZ\tGraham County\tH1\n85530\t4009\tBylas\tAZ\tGraham County\tH1\n85534\t4011\tDuncan\tAZ\tGreenlee County\tH1\n85540\t4011\tMorenci\tAZ\tGreenlee County\tH1\n85533\t4011\tClifton\tAZ\tGreenlee County\tH1\n85922\t4011\tBlue\tAZ\tGreenlee County\tH1\n85359\t4012\tQuartzsite\tAZ\tLa Paz County\tH1\n85328\t4012\tCibola\tAZ\tLa Paz County\tH1\n85325\t4012\tBouse\tAZ\tLa Paz County\tH1\n85357\t4012\tWenden\tAZ\tLa Paz County\tH1\n85348\t4012\tSalome\tAZ\tLa Paz County\tH1\n85346\t4012\tQuartzsite\tAZ\tLa Paz County\tH1\n85334\t4012\tEhrenberg\tAZ\tLa Paz County\tH1\n85344\t4012\tParker\tAZ\tLa Paz County\tH1\n85040\t4013\tPhoenix\tAZ\tMaricopa County\tH1\n85031\t4013\tPhoenix\tAZ\tMaricopa County\tH1\n85045\t4013\tPhoenix\tAZ\tMaricopa County\tH1\n85023\t4013\tPhoenix\tAZ\tMaricopa County\tH1\n85054\t4013\tPhoenix\tAZ\tMaricopa County\tH1\n85201\t4013\tMesa\tAZ\tMaricopa County\tH1\n85210\t4013\tMesa\tAZ\tMaricopa County\tH1\n85255\t4013\tScottsdale\tAZ\tMaricopa County\tH1\n85263\t4013\tRio verde\tAZ\tMaricopa County\tH1\n85004\t4013\tPhoenix\tAZ\tMaricopa County\tH1\n85006\t4013\tPhoenix\tAZ\tMaricopa County\tH1\n85011\t4013\tPhoenix\tAZ\tMaricopa County\tH1\n85286\t4013\tChandler\tAZ\tMaricopa County\tH1\n85295\t4013\tGilbert\tAZ\tMaricopa County\tH1\n85308\t4013\tGlendale\tAZ\tMaricopa County\tH1\n85283\t4013\tTempe\tAZ\tMaricopa County\tH1\n85388\t4013\tSurprise\tAZ\tMaricopa County\tH1\n85312\t4013\tGlendale\tAZ\tMaricopa County\tH1\n85343\t4013\tPalo verde\tAZ\tMaricopa County\tH1\n85119\t4013\tApache junction\tAZ\tMaricopa County\tH1\n85087\t4013\tNew river\tAZ\tMaricopa County\tH1\n85063\t4013\tPhoenix\tAZ\tMaricopa County\tH1\n85060\t4013\tPhoenix\tAZ\tMaricopa County\tH1\n85139\t4013\tMaricopa\tAZ\tMaricopa County\tH1\n85120\t4013\tApache junction\tAZ\tMaricopa County\tH1\n85233\t4013\tGilbert\tAZ\tMaricopa County\tH1\n85260\t4013\tScottsdale\tAZ\tMaricopa County\tH1\n85246\t4013\tChandler\tAZ\tMaricopa County\tH1\n85016\t4013\tPhoenix\tAZ\tMaricopa County\tH1\n85019\t4013\tPhoenix\tAZ\tMaricopa County\tH1\n85302\t4013\tGlendale\tAZ\tMaricopa County\tH1\n85304\t4013\tGlendale\tAZ\tMaricopa County\tH1\n85303\t4013\tGlendale\tAZ\tMaricopa County\tH1\n85337\t4013\tGila bend\tAZ\tMaricopa County\tH1\n85323\t4013\tAvondale\tAZ\tMaricopa County\tH1\n85329\t4013\tCashion\tAZ\tMaricopa County\tH1\n85351\t4013\tSun city\tAZ\tMaricopa County\tH1\n85387\t4013\tSurprise\tAZ\tMaricopa County\tH1\n85001\t4013\tPhoenix\tAZ\tMaricopa County\tH1\n85211\t4013\tMesa\tAZ\tMaricopa County\tH1\n85380\t4013\tPeoria\tAZ\tMaricopa County\tH1\n85277\t4013\tMesa\tAZ\tMaricopa County\tH1\n85121\t4013\tBapchule\tAZ\tMaricopa County\tH1\n85024\t4013\tPhoenix\tAZ\tMaricopa County\tH1\n85022\t4013\tPhoenix\tAZ\tMaricopa County\tH1\n85203\t4013\tMesa\tAZ\tMaricopa County\tH1\n85208\t4013\tMesa\tAZ\tMaricopa County\tH1\n85253\t4013\tParadise valley\tAZ\tMaricopa County\tH1\n85254\t4013\tScottsdale\tAZ\tMaricopa County\tH1\n85268\t4013\tFountain hills\tAZ\tMaricopa County\tH1\n85282\t4013\tTempe\tAZ\tMaricopa County\tH1\n85310\t4013\tGlendale\tAZ\tMaricopa County\tH1\n85311\t4013\tGlendale\tAZ\tMaricopa County\tH1\n85307\t4013\tGlendale\tAZ\tMaricopa County\tH1\n85331\t4013\tCave creek\tAZ\tMaricopa County\tH1\n85327\t4013\tCave creek\tAZ\tMaricopa County\tH1\n85333\t4013\tDateland\tAZ\tMaricopa County\tH1\n85361\t4013\tWittmann\tAZ\tMaricopa County\tH1\n85396\t4013\tBuckeye\tAZ\tMaricopa County\tH1\n85381\t4013\tPeoria\tAZ\tMaricopa County\tH1\n85355\t4013\tWaddell\tAZ\tMaricopa County\tH1\n85545\t4013\tRoosevelt\tAZ\tMaricopa County\tH1\n85074\t4013\tPhoenix\tAZ\tMaricopa County\tH1\n85035\t4013\tPhoenix\tAZ\tMaricopa County\tH1\n85048\t4013\tPhoenix\tAZ\tMaricopa County\tH1\n85021\t4013\tPhoenix\tAZ\tMaricopa County\tH1\n85042\t4013\tPhoenix\tAZ\tMaricopa County\tH1\n85079\t4013\tPhoenix\tAZ\tMaricopa County\tH1\n85070\t4013\tPhoenix\tAZ\tMaricopa County\tH1\n85202\t4013\tMesa\tAZ\tMaricopa County\tH1\n85142\t4013\tQueen creek\tAZ\tMaricopa County\tH1\n85205\t4013\tMesa\tAZ\tMaricopa County\tH1\n85257\t4013\tScottsdale\tAZ\tMaricopa County\tH1\n85215\t4013\tMesa\tAZ\tMaricopa County\tH1\n85225\t4013\tChandler\tAZ\tMaricopa County\tH1\n85214\t4013\tMesa\tAZ\tMaricopa County\tH1\n85008\t4013\tPhoenix\tAZ\tMaricopa County\tH1\n85017\t4013\tPhoenix\tAZ\tMaricopa County\tH1\n85020\t4013\tPhoenix\tAZ\tMaricopa County\tH1\n85299\t4013\tGilbert\tAZ\tMaricopa County\tH1\n85269\t4013\tFountain hills\tAZ\tMaricopa County\tH1\n85375\t4013\tSun city west\tAZ\tMaricopa County\tH1\n85392\t4013\tAvondale\tAZ\tMaricopa County\tH1\n85395\t4013\tGoodyear\tAZ\tMaricopa County\tH1\n85285\t4013\tTempe\tAZ\tMaricopa County\tH1\n85076\t4013\tPhoenix\tAZ\tMaricopa County\tH1\n85030\t4013\tPhoenix\tAZ\tMaricopa County\tH1\n85043\t4013\tPhoenix\tAZ\tMaricopa County\tH1\n85086\t4013\tPhoenix\tAZ\tMaricopa County\tH1\n85066\t4013\tPhoenix\tAZ\tMaricopa County\tH1\n85068\t4013\tPhoenix\tAZ\tMaricopa County\tH1\n85053\t4013\tPhoenix\tAZ\tMaricopa County\tH1\n85082\t4013\tPhoenix\tAZ\tMaricopa County\tH1\n85249\t4013\tChandler\tAZ\tMaricopa County\tH1\n85226\t4013\tChandler\tAZ\tMaricopa County\tH1\n85266\t4013\tScottsdale\tAZ\tMaricopa County\tH1\n85258\t4013\tScottsdale\tAZ\tMaricopa County\tH1\n85264\t4013\tFort mcdowell\tAZ\tMaricopa County\tH1\n85003\t4013\tPhoenix\tAZ\tMaricopa County\tH1\n85014\t4013\tPhoenix\tAZ\tMaricopa County\tH1\n85005\t4013\tPhoenix\tAZ\tMaricopa County\tH1\n85284\t4013\tTempe\tAZ\tMaricopa County\tH1\n85281\t4013\tTempe\tAZ\tMaricopa County\tH1\n85326\t4013\tBuckeye\tAZ\tMaricopa County\tH1\n85363\t4013\tYoungtown\tAZ\tMaricopa County\tH1\n85373\t4013\tSun city\tAZ\tMaricopa County\tH1\n85340\t4013\tLitchfield park\tAZ\tMaricopa County\tH1\n85345\t4013\tPeoria\tAZ\tMaricopa County\tH1\n85374\t4013\tSurprise\tAZ\tMaricopa County\tH1\n85382\t4013\tPeoria\tAZ\tMaricopa County\tH1\n85390\t4013\tWickenburg\tAZ\tMaricopa County\tH1\n85342\t4013\tMorristown\tAZ\tMaricopa County\tH1\n85318\t4013\tGlendale\tAZ\tMaricopa County\tH1\n85252\t4013\tScottsdale\tAZ\tMaricopa County\tH1\n85236\t4013\tHigley\tAZ\tMaricopa County\tH1\n85244\t4013\tChandler\tAZ\tMaricopa County\tH1\n85271\t4013\tScottsdale\tAZ\tMaricopa County\tH1\n85037\t4013\tPhoenix\tAZ\tMaricopa County\tH1\n85051\t4013\tPhoenix\tAZ\tMaricopa County\tH1\n85212\t4013\tMesa\tAZ\tMaricopa County\tH1\n85207\t4013\tMesa\tAZ\tMaricopa County\tH1\n85206\t4013\tMesa\tAZ\tMaricopa County\tH1\n85234\t4013\tGilbert\tAZ\tMaricopa County\tH1\n85248\t4013\tChandler\tAZ\tMaricopa County\tH1\n85224\t4013\tChandler\tAZ\tMaricopa County\tH1\n85216\t4013\tMesa\tAZ\tMaricopa County\tH1\n85262\t4013\tScottsdale\tAZ\tMaricopa County\tH1\n85259\t4013\tScottsdale\tAZ\tMaricopa County\tH1\n85267\t4013\tScottsdale\tAZ\tMaricopa County\tH1\n85009\t4013\tPhoenix\tAZ\tMaricopa County\tH1\n85296\t4013\tGilbert\tAZ\tMaricopa County\tH1\n85297\t4013\tGilbert\tAZ\tMaricopa County\tH1\n85305\t4013\tGlendale\tAZ\tMaricopa County\tH1\n85309\t4013\tLuke air force base\tAZ\tMaricopa County\tH1\n85280\t4013\tTempe\tAZ\tMaricopa County\tH1\n85379\t4013\tSurprise\tAZ\tMaricopa County\tH1\n85275\t4013\tMesa\tAZ\tMaricopa County\tH1\n85376\t4013\tSun city west\tAZ\tMaricopa County\tH1\n85061\t4013\tPhoenix\tAZ\tMaricopa County\tH1\n85026\t4013\tPhoenix\tAZ\tMaricopa County\tH1\n85320\t4013\tAguila\tAZ\tMaricopa County\tH1\n85147\t4013\tSacaton\tAZ\tMaricopa County\tH1\n85032\t4013\tPhoenix\tAZ\tMaricopa County\tH1\n85044\t4013\tPhoenix\tAZ\tMaricopa County\tH1\n85027\t4013\tPhoenix\tAZ\tMaricopa County\tH1\n85034\t4013\tPhoenix\tAZ\tMaricopa County\tH1\n85083\t4013\tPhoenix\tAZ\tMaricopa County\tH1\n85085\t4013\tPhoenix\tAZ\tMaricopa County\tH1\n85029\t4013\tPhoenix\tAZ\tMaricopa County\tH1\n85028\t4013\tPhoenix\tAZ\tMaricopa County\tH1\n85067\t4013\tPhoenix\tAZ\tMaricopa County\tH1\n85204\t4013\tMesa\tAZ\tMaricopa County\tH1\n85251\t4013\tScottsdale\tAZ\tMaricopa County\tH1\n85256\t4013\tScottsdale\tAZ\tMaricopa County\t
